vi "Test Find Readers of Data -- NEEDS CLEANUP.vi"   [LabVIEW 2020]
uses:
  source/JKI SM/JKI SM.lvclass
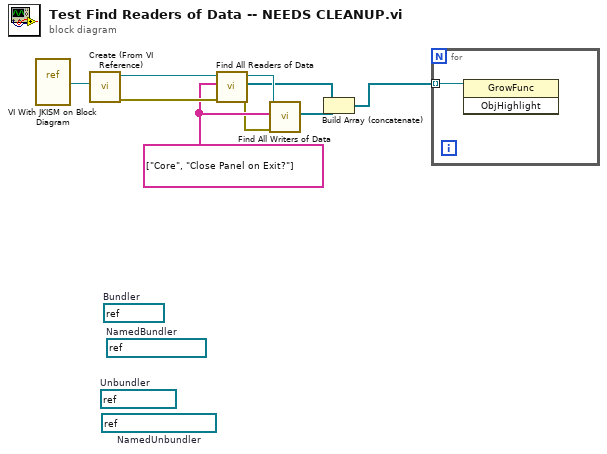
[diagram p0: block diagram]
diagram:
  w6 = string[] ["Core", "Close Panel on Exit?"] ("Full Element Name")
  (unwired) refnum<vi> refnum  # Unbundler
  (unwired) refnum<vi> refnum  # Bundler
  (unwired) refnum<vi> refnum  # NamedUnbundler
  (unwired) refnum<vi> refnum  # NamedBundler
  n1 = vi-ref "VI With JKISM on Block Diagram.vi"() -> (w9:refnum<vi>)
  n2 = call "Create (From VI Reference).vi"("VI"=w9) -> ("error out"=w7:errorcluster, "JKI SM out"=w8:refnum<class "JKI SM.lvclass">)  [unwired: 9 in]
  n3 = call "Find All Readers of Data.vi"("error in (no error)"=w7, "Full Element Name"=w6, "JKI SM in"=w8) -> ("error out"=w4:errorcluster, "NamedUnbundlers"=w2:refnum<vi>[], "JKI SM out"=w5:refnum<class "JKI SM.lvclass">)  [unwired: 6 in]
  n4 = call "Find All Writers of Data.vi"("error in (no error)"=w4, "Full Element Name"=w6, "JKI SM in"=w5) -> ("NamedBundlers"=w3:refnum<vi>[])  [unwired: 5 in, 3 out]
  n5 = Build Array (concatenate)(w2, w3) -> (w1:refnum<vi>[])
  n6 = for {
    tunnel: w1 -> [w10] mode=indexing
    n7 = invoke class="GrowFunc" method="ObjHighlight"(reference=w10) -> ()  [unwired: 2 in, 3 out]
  }
